vi "INTERFAZ.vi"() -> ()   [LabVIEW 2021]
uses:
  <vilib>/Instr/_visa.llb/Select Event Type.ctl
  <vilib>/Instr/_visa.llb/VISA Configure Serial Port (Instr).vi
panel:
  in  "Stop 2":bool
  out "?":dbl
  out "?":dbl
  out "?":dbl
  in  "?":refnum<visa-resource-name>
  in  "Stop":bool
  out "Waveform Chart 2":dbl(graph)
  out "Vertical Pointer Slide":dbl(slide) scale=0.0..100.0
  out "?":dbl(graph)
  out "Waveform Chart":dbl(graph)
  out "PESO":i32(slide) scale=0.0..100.0
  in  "ENVIAR\nENVIAR":bool
  out "NIVEL":dbl(slide) scale=0.0..100.0
  # "PANEL DE CONTROL"
  # "PESO"
  # "TEMPERATURA"
  # "NIVEL"
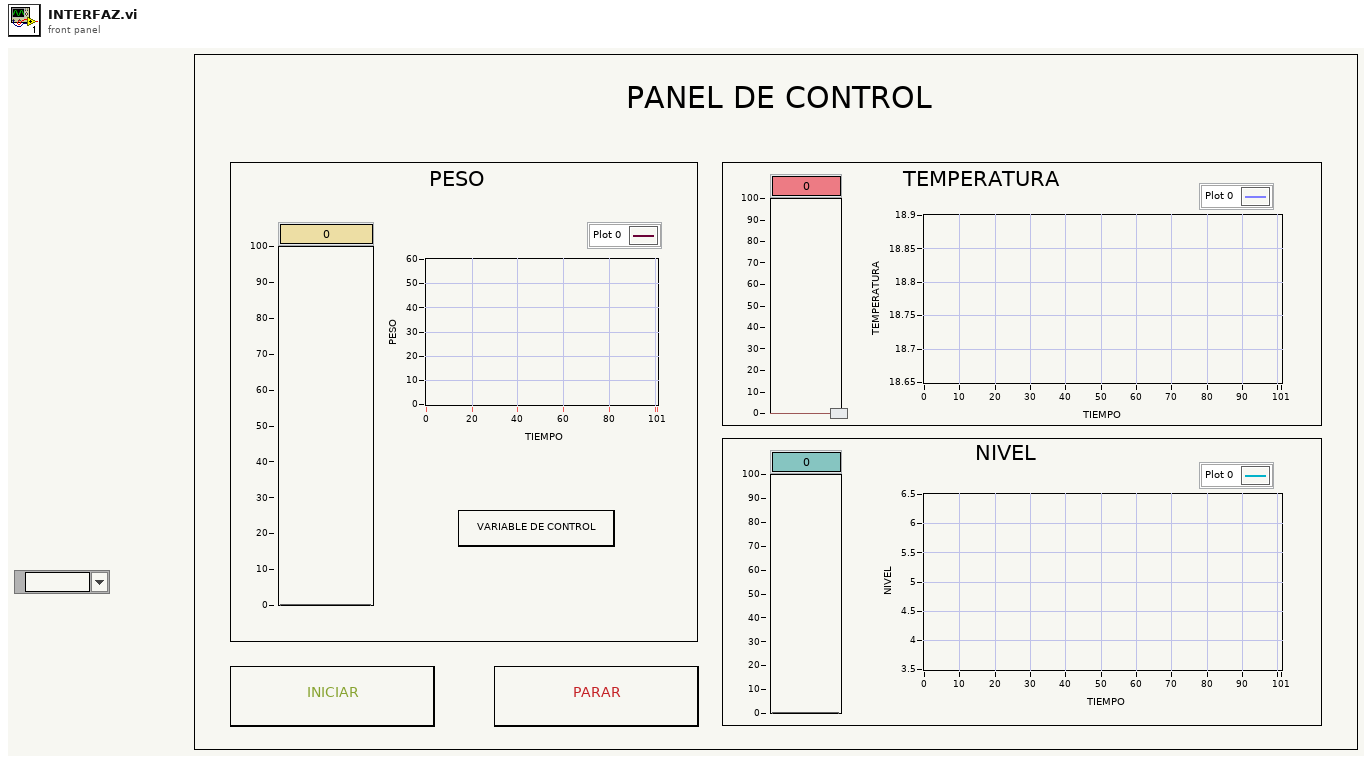
[diagram p1: front panel]
types:
  T1 = typedef "Select Event Type.ctl" = u32
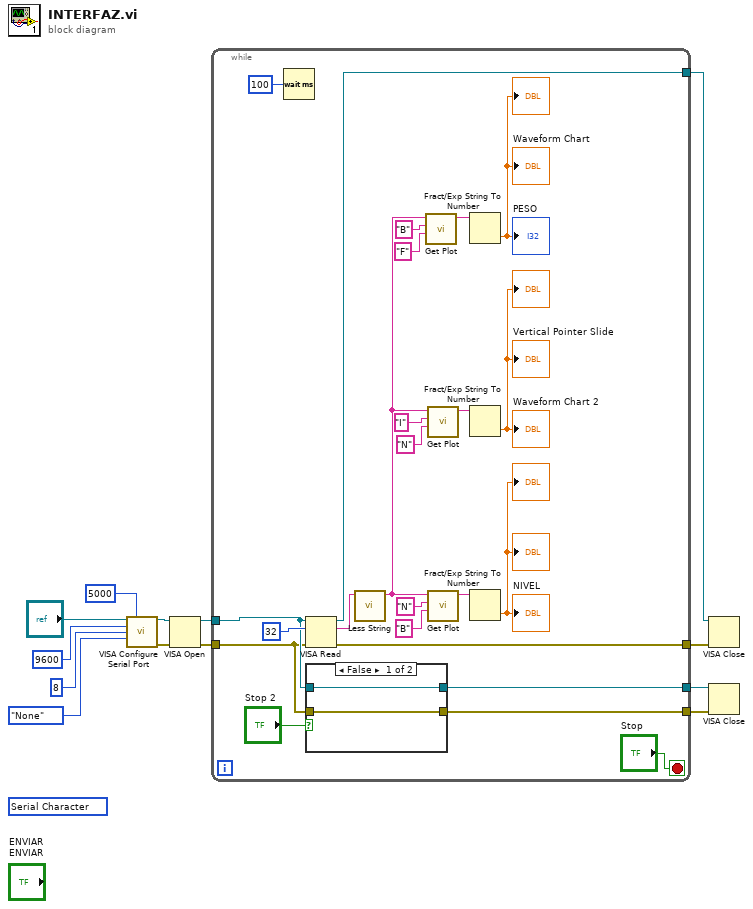
[diagram p0: block diagram]
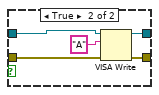
[diagram p2: hidden frame]
diagram:
  (unwired) T1 1073684533 items=["Service Request"=1073684491, "Trigger"=3221168138, "Clear"=1073684493, "VXI Signal"=1073684512, "VXI/VME Interrupt"=3221168161, "VXI/VME Sysfail"=1073684509, "VXI/VME Sysreset"=1073684510, "GPIB CIC"=1073684498, "GPIB Talk"=1073684499, "GPIB Listen"=1073684500, "PXI Interrupt"=1073684514, "Serial Break"=1073684515, "Serial TermChar"=1073684516, "Serial CTS"=1073684521, "Serial DSR"=1073684522, "Serial DCD"=1073684524, "Serial RI"=1073684526, "Serial Character"=1073684533, "USB Interrupt"=1073684535, "All Enabled"=1073709055] ("Event Type")
  n1 = call-poly "VISA Configure Serial Port"("VISA resource name"="?", "timeout (10sec)"=u32 5000, "baud rate (9600)"=u32 9600, "data bits (8)"=u16 8, "parity (0:none)"=enum16{"None", "Odd", "Even", "Mark", "Space"}."None") -> ("VISA resource name out"=w4:refnum<visa-resource-name>, "error out"=w3:errorcluster)  [unwired: 9 in]
  n2 = VISA Open(error in (no error)=w3, VISA resource name=w4) -> (VISA resource name=w2:refnum<visa-resource-name>, error out=w1:errorcluster)  [unwired: 3 in]
  n3 = while {
    tunnel: [w35] -> w13
    tunnel: [w36] -> w12
    tunnel: [w34] -> w11
    tunnel: [w33] -> w10
    tunnel: w2 -> [w30]
    tunnel: w1 -> [w29]
    stop <- "Stop" stop-if-true
    n4 = Wait (ms)(milliseconds to wait=u32 100) -> ()  [unwired: 1 out]
    n5 = VISA Read(VISA resource name=w30, byte count=u32 32, error in (no error)=w29) -> (VISA resource name out=w35:refnum<visa-resource-name>, read buffer=w28:string, error out=w36:errorcluster)  [unwired: 1 out]
    n6 = case shown="False" "Stop 2" {
      tunnel: w30 -> [w39 w44]
      tunnel: w29 -> [w38 w43]
      tunnel: [w39 w42] -> w34
      tunnel: [w38 w41] -> w33
      frame False {
      }
      frame True {
        n7 = VISA Write(VISA resource name=w44, write buffer="A", error in (no error)=w43) -> (VISA resource name out=w42:refnum<visa-resource-name>, error out=w41:errorcluster)  [unwired: 1 out]
      }
    }
    n8 = call "Less String.vi"("Input String"=w28) -> ("Out String"=w23:string)  [unwired: 10 in]
    n9 = call "Get Plot.vi"("Stop"="F", "Start"="B", "Input String"=w23) -> ("Out String"=w20:string)  [unwired: 8 in]
    n10 = call "Get Plot.vi"("Stop"="N", "Start"="I", "Input String"=w23) -> ("Out String"=w18:string)  [unwired: 8 in]
    n11 = call "Get Plot.vi"("Stop"="B", "Start"="N", "Input String"=w23) -> ("Out String"=w16:string)  [unwired: 8 in]
    n12 = Fract/Exp String To Number(string=w20) -> (number=→"?" →"Waveform Chart" →"PESO":dbl)  [unwired: 3 in, 1 out]
    n13 = Fract/Exp String To Number(string=w18) -> (number=→"Vertical Pointer Slide" →"Waveform Chart 2" →"?":dbl)  [unwired: 3 in, 1 out]
    n14 = Fract/Exp String To Number(string=w16) -> (number=→"NIVEL" →"?" →"?":dbl)  [unwired: 3 in, 1 out]
  }
  n15 = VISA Close(VISA resource name=w13, error in (no error)=w12) -> ()  [unwired: 1 out]
  n16 = VISA Close(VISA resource name=w11, error in (no error)=w10) -> ()  [unwired: 1 out]
